vi "split 2 sequence array.vi"(10 "Enum":enum16{"columns", "rows"}(ring)=enum."rows", 11 "2 sequence array":dbl[][](array[numeric])) -> (2 "i1 sequence":dbl[](array[numeric]), 3 "i0 sequence":dbl[](array[numeric]))   [LabVIEW 2018]
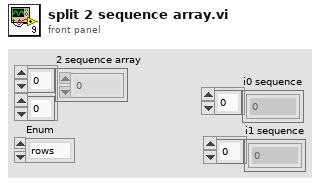
[diagram p1: front panel]
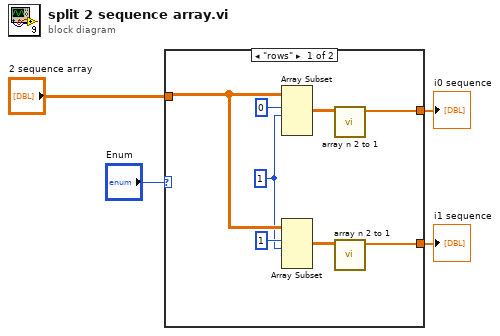
[diagram p0: block diagram]
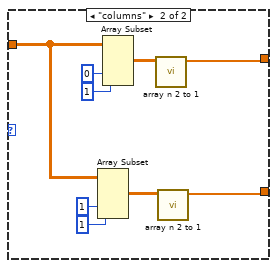
[diagram p2: hidden frame]
diagram:
  n1 = case shown="\"rows\"" "Enum" {
    tunnel: "2 sequence array" -> [w10 w15]
    tunnel: [w6 w14] -> w2
    tunnel: [w5 w13] -> w1
    frame "rows" {
      w7 = 1 ("length")
      n2 = Array Subset(array=w10, index (row)=0 ("index"), length (row)=w7) -> (w12:dbl[][])  [unwired: 2 in]
      n3 = Array Subset(array=w10, index (row)=1 ("index"), length (row)=w7) -> (w11:dbl[][])  [unwired: 2 in]
      n4 = call "array n 2 to 1.vi"("2N array"=w12) -> ("1N array"=w6:dbl[])  [unwired: 10 in]
      n5 = call "array n 2 to 1.vi"("2N array"=w11) -> ("1N array"=w5:dbl[])  [unwired: 10 in]
    }
    frame "columns" {
      n6 = Array Subset(array=w15, index (col)=1 ("index"), length (col)=1 ("length")) -> (w16:dbl[][])  [unwired: 2 in]
      n7 = Array Subset(array=w15, index (col)=0 ("index"), length (col)=1 ("length")) -> (w17:dbl[][])  [unwired: 2 in]
      n8 = call "array n 2 to 1.vi"("2N array"=w17) -> ("1N array"=w14:dbl[])  [unwired: 10 in]
      n9 = call "array n 2 to 1.vi"("2N array"=w16) -> ("1N array"=w13:dbl[])  [unwired: 10 in]
    }
  }
  "i0 sequence" <- w2
  "i1 sequence" <- w1
